vi "testTimestampParsingZ.vi"(8 "error in (no error)":errorcluster, 11 "TestCase in":refnum<class "EasyXMLTest.lvclass">) -> (0 "error out":errorcluster, 3 "TestCase out":refnum<class "EasyXMLTest.lvclass">)   [LabVIEW 2013, in "EasyXMLTest.lvclass"]
doc: "Verify that error in is not overwritten"
uses:
  EasyXMLTest.lvclass
panel:
  out "dateTime out":timestamp
  out "Produced Data":variant
  out "Expected Data":variant
  out "XML String":string
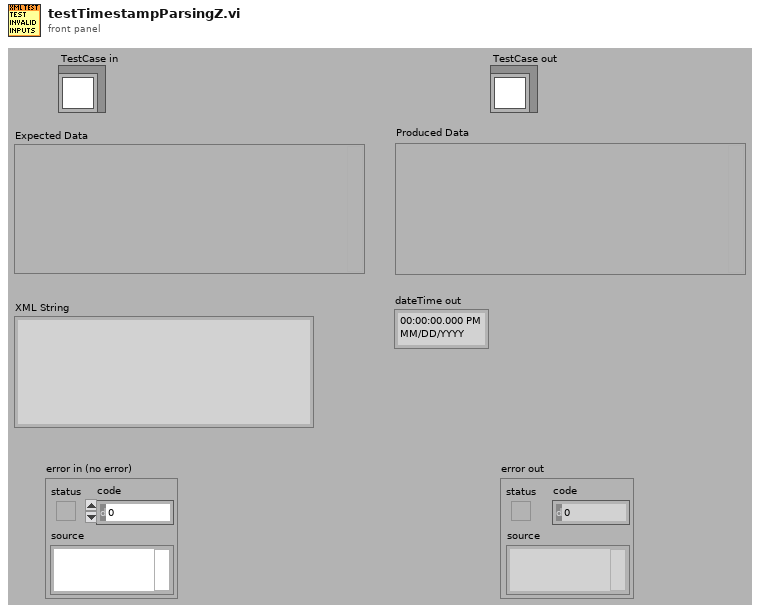
[diagram p1: front panel]
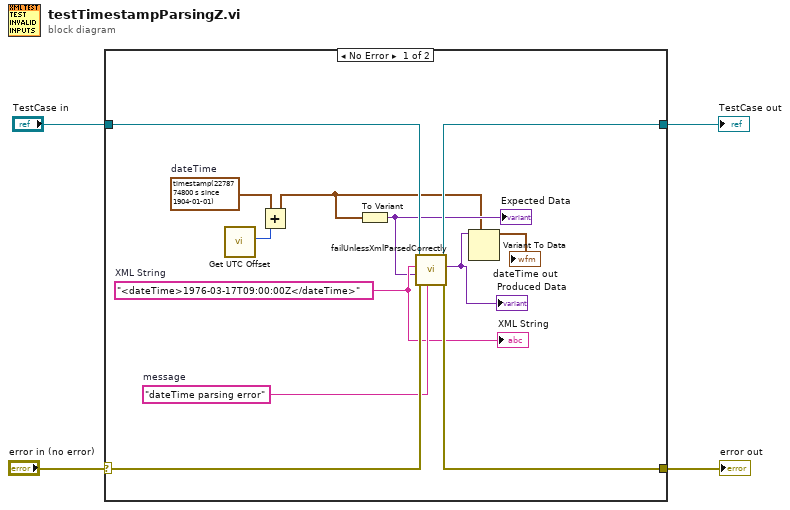
[diagram p0: block diagram]
diagram:
  n1 = case shown="No Error" "error in (no error)" {
    selector: "error in (no error)" -> [w15 w18]
    tunnel: [w14 w18] -> w2
    tunnel: [w13 w17] -> w1
    tunnel: "TestCase in" -> [w16 w17]
    frame No Error {
      w6 = timestamp(2278774800 s since 1904-01-01)  # dateTime
      w11 = "<dateTime>1976-03-17T09:00:00Z</dateTime>"  # XML String
      w12 = "dateTime parsing error"  # message
      n2 = call "Get UTC Offset.vi"() -> ("UTC Offset (seconds)"=w7:i32)  [unwired: 10 in, 1 out]
      n3 = Add(x=w6, y=w7) -> (x+y=w5:timestamp)
      n4 = To Variant(anything=w5) -> (Variant=w10:variant)
      "Expected Data" <- w10
      n5 = call "failUnlessXmlParsedCorrectly.vi"("message (\"\")"=w12, "error in"=w15, "Expected Data"=w10, "XML String"=w11, "reference in"=w16) -> ("error out"=w14:errorcluster, "Produced Data"=w9:variant, "reference in"=w13:refnum<class "EasyXMLTest.lvclass">)  [unwired: 4 in]
      "Produced Data" <- w9
      n6 = Variant To Data(type=w5, Variant=w9) -> (data=→"dateTime out":timestamp)  [unwired: 1 in, 1 out]
      "XML String" <- w11
    }
    frame Error {
    }
  }
  "error out" <- w2
  "TestCase out" <- w1
